vi "IV Keithley 2400 SVI - Sweep.vi"(3 "Number of Points (5)":u32=5, 4 "Manual Range (1.0)":dbl=1.0, 5 "Maximum Amplitude (2)":dbl=2.0, 6 "Enable Auto Range (T:Enable)":bool=TRUE, 7 "Minimum Amplitude (1)":dbl=1.0, 8 "error in (no error)":errorcluster, 9 "Timeout (10000 ms)":i32=10000 format="%#.6g", 10 "Manual Settling Delay (0 sec)":dbl, 11 "VISA resource name":refnum<visa-resource-name>="GPIB0::23::INSTR") -> (0 "error out":errorcluster, 1 "Current":sgl[](array[numeric]), 2 "Voltage":sgl[](array[numeric]))   [LabVIEW 2011]
doc: "Configures a sweep and takes voltage and current readings at each point."
uses:
  <instrlib>/Keithley 24XX/Public/Data/Read (Multiple Points).vi
  <instrlib>/Keithley 24XX/Keithley 24XX.lvlib
panel:
  out "Waveform Graph":sgl[][](graph)
  # "(c) 2006 National Instruments.  ALL RIGHTS RESERVED."
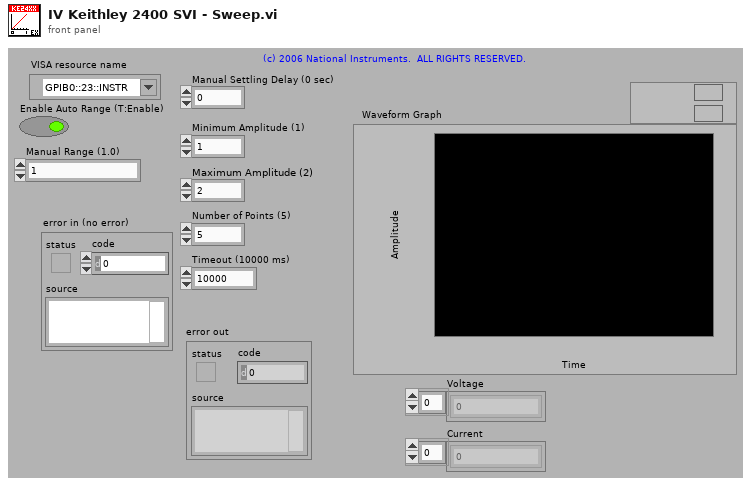
[diagram p1: front panel]
types:
  T1 = cluster{"Baud Rate":u32, "Parity":u16, "Data Bits":u16, "Stop Bits":u16, "Flow Control":u16}
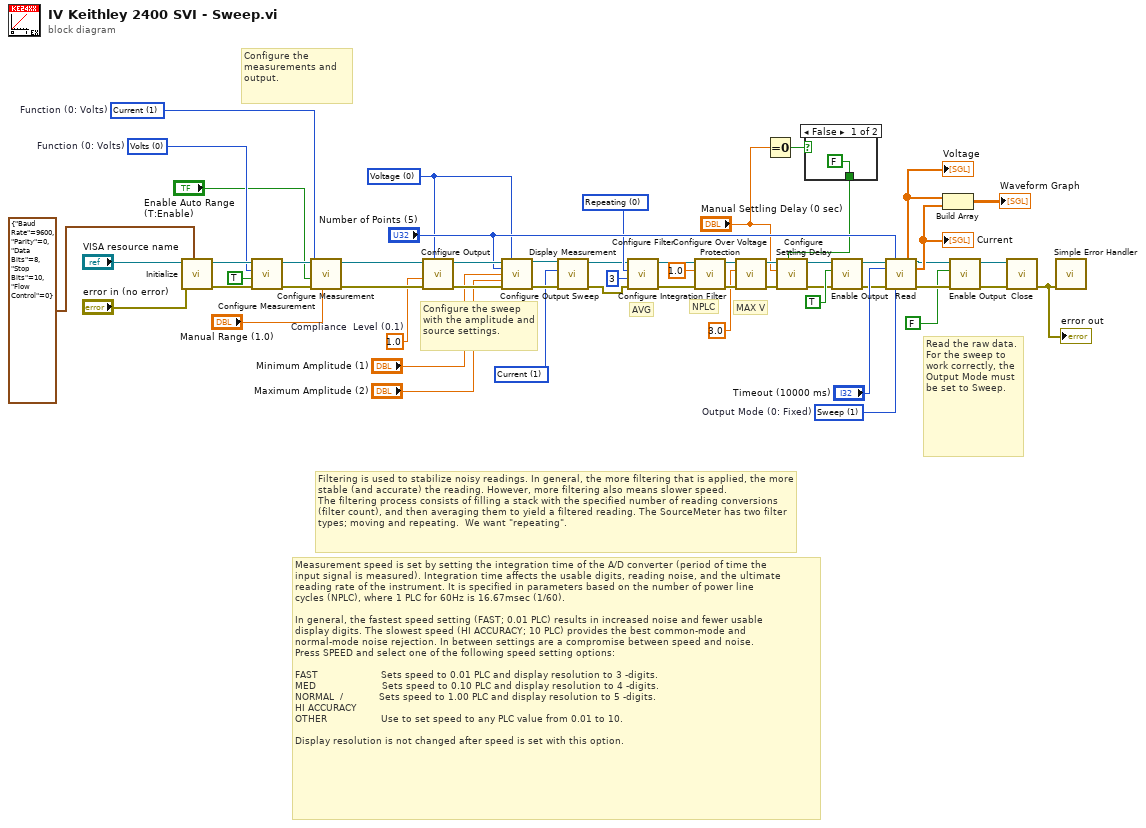
[diagram p0: block diagram]
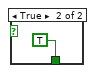
[diagram p2: hidden frame]
diagram:
  w1 = u16 1 items=["Voltage", "Current", "Resistance"] ("Displayed Measurement (0: Voltage)")
  w29 = 1.0  # Compliance  Level (0.1)
  w24 = u16 0 items=["Voltage", "Current"] ("Source Mode  (0: Voltage)")
  w19 = u16 0 items=["Repeating", "Moving"] ("Filter Type  (0: Repeating)")
  w27 = u16 1 items=["Volts", "Current", "Resistance"]  # Function (0: Volts)
  w28 = u16 0 items=["Volts", "Current", "Resistance"]  # Function (0: Volts)
  w38 = u16 1 items=["Fixed", "Sweep", "List"]  # Output Mode (0: Fixed)
  # "Measurement speed is set by setting the integration time of the A/D converter (period of time the\ninput signal is measured). Integration time affects the usable digits, reading noise, and the ultimate\nreading rate of the instrument. It is specified in parameters based on the number of power line\ncycles (NPLC), where 1 PLC for 60Hz is 16.67msec (1/60).\n\nIn general, the fastest speed setting (FAST; 0.01 PLC) results in increased noise and fewer usable\ndisplay digits. The slowest speed (HI ACCURACY; 10 PLC) provides the best common-mode and\nnormal-mode noise rejection. In between settings are a compromise between speed and noise.\nPress SPEED and select one of the following speed setting options:\n\nFAST                     Sets speed to 0.01 PLC and display resolution to 3 -digits.\nMED                      Sets speed to 0.10 PLC and display resolution to 4 -digits.\nNORMAL  /            Sets speed to 1.00 PLC and display resolution to 5 -digits.\nHI ACCURACY     \nOTHER                  Use to set speed to any PLC value from 0.01 to 10.\n\nDisplay resolution is not changed after speed is set with this option."
  # "Filtering is used to stabilize noisy readings. In general, the more filtering that is applied, the more stable (and accurate) the reading. However, more filtering also means slower speed.\nThe filtering process consists of filling a stack with the specified number of reading conversions (filter count), and then averaging them to yield a filtered reading. The SourceMeter has two filter types; moving and repeating.  We want \"repeating\"."
  # "MAX V"
  # "AVG"
  # "NPLC"
  # "Read the raw data.  For the sweep to work correctly, the Output Mode must be set to Sweep."
  # "Configure the sweep with the amplitude and source settings."
  # "Configure the measurements and output."
  n1 = call <instrlib>:"Initialize.vi"("Serial Configuration"=T1 {"Baud Rate"=9600, "Parity"=0, "Data Bits"=8, "Stop Bits"=10, "Flow Control"=0}, "error in (no error)"="error in (no error)", "VISA resource name"="VISA resource name") -> ("error out"=w54:errorcluster, "VISA resource name out"=w55:refnum<visa-resource-name>)  [unwired: 7 in]
  n2 = call <instrlib>:"Configure Measurement.vi"("error in (no error)"=w54, "Enable Auto Range (T:Enable)"=TRUE, "Function (0: Volts)"=w28, "VISA resource name"=w55) -> ("error out"=w53:errorcluster, "VISA resource name out"=w52:refnum<visa-resource-name>)  [unwired: 6 in]
  n3 = call <instrlib>:"Configure Measurement.vi"("Manual Range (1.0)"="Manual Range (1.0)", "error in (no error)"=w53, "Enable Auto Range (T:Enable)"="Enable Auto Range (T:Enable)", "Function (0: Volts)"=w27, "VISA resource name"=w52) -> ("error out"=w50:errorcluster, "VISA resource name out"=w51:refnum<visa-resource-name>)  [unwired: 5 in]
  n4 = call <instrlib>:"Configure Output.vi"("Source Mode  (0: Voltage)"=w24, "error in (no error)"=w50, "Compliance  Level (0.1)"=w29, "VISA resource name"=w51) -> ("error out"=w49:errorcluster, "VISA resource name out"=w48:refnum<visa-resource-name>)  [unwired: 6 in]
  n5 = call <instrlib>:"Configure Output Sweep.vi"("VISA resource name"=w48, "Source Mode  (0: Voltage)"=w24, "Number of Points (5)"="Number of Points (5)", "Minimum Amplitude (1)"="Minimum Amplitude (1)", "Maximum Amplitude (2)"="Maximum Amplitude (2)", "error in (no error)"=w49) -> ("VISA resource name out"=w4:refnum<visa-resource-name>, "error out"=w5:errorcluster)  [unwired: 8 in]
  n6 = call <instrlib>:"Display Measurement.vi"("error in (no error)"=w5, "Displayed Measurement (0: Voltage)"=w1, "VISA resource name"=w4) -> ("error out"=w2:errorcluster, "VISA resource name out"=w3:refnum<visa-resource-name>)  [unwired: 7 in]
  n7 = call <instrlib>:"Configure Filter.vi"("error in (no error)"=w2, "Number of Filter Readings (3)"=u32 3, "Filter Type  (0: Repeating)"=w19, "VISA resource name"=w3) -> ("error out"=w20:errorcluster, "VISA resource name out"=w21:refnum<visa-resource-name>)  [unwired: 6 in]
  n8 = call <instrlib>:"Configure Integration Filter.vi"("error in (no error)"=w20, "Measurement Speed (1 PLC)"=1.0, "VISA resource name"=w21) -> ("error out"=w14:errorcluster, "VISA resource name out"=w16:refnum<visa-resource-name>)  [unwired: 7 in]
  n9 = call <instrlib>:"Configure Over Voltage Protection.vi"("error in (no error)"=w14, "Voltage Limit (0.0 V)"=3.0, "VISA resource name"=w16) -> ("error out"=w13:errorcluster, "VISA resource name out"=w15:refnum<visa-resource-name>)  [unwired: 7 in]
  n10 = Equal To 0?(x="Manual Settling Delay (0 sec)") -> (x = 0?=w8:bool)
  n11 = case shown="False" w8 {
    tunnel: [FALSE ("Auto Settle (T: Enable)") TRUE ("Auto Settle (T: Enable)")] -> w6
    frame False {
    }
    frame True {
    }
  }
  n12 = call <instrlib>:"Configure Settling Delay.vi"("Auto Settle (T: Enable)"=w6, "error in (no error)"=w13, "Manual Settling Delay (0 sec)"="Manual Settling Delay (0 sec)", "VISA resource name"=w15) -> ("error out"=w23:errorcluster, "VISA resource name out"=w22:refnum<visa-resource-name>)  [unwired: 6 in]
  n13 = call <instrlib>:"Enable Output.vi"("error in (no error)"=w23, "Enable Output (T: Enable)"=TRUE, "VISA resource name"=w22) -> ("error out"=w31:errorcluster, "VISA resource name out"=w30:refnum<visa-resource-name>)  [unwired: 7 in]
  n14 = call-poly <instrlib>:"Read.vi"("VISA resource name"=w30, "Sample Count (1)"="Number of Points (5)", "Timeout (10000 ms)"="Timeout (10000 ms)", "error in (no error)"=w31, "Output Mode (0: Fixed)"=w38) -> ("Voltage"=w43:sgl[], "VISA resource name out"=w33:refnum<visa-resource-name>, "Current"=w42:sgl[], "error out"=w34:errorcluster)  [unwired: 4 in, 3 out]
  "Voltage" <- w43
  "Current" <- w42
  n15 = Build Array(w43, w42) -> (→"Waveform Graph":sgl[][])
  n16 = call <instrlib>:"Enable Output.vi"("error in (no error)"=w34, "Enable Output (T: Enable)"=FALSE, "VISA resource name"=w33) -> ("error out"=w35:errorcluster, "VISA resource name out"=w36:refnum<visa-resource-name>)  [unwired: 7 in]
  n17 = call <instrlib>:"Close.vi"("error in (no error)"=w35, "VISA resource name"=w36) -> ("error out"=w37:errorcluster)  [unwired: 9 in]
  "error out" <- w37
  n18 = call <vilib>:"Simple Error Handler.vi"("error in (no error)"=w37) -> ()  [unwired: 4 in, 5 out]
